vi "fpga_FIFO control (M Class_50Hz).vi"(0 "Time stamp":fxp<+,64,32> format="%.42g", 1 "reset":bool, 2 "filter delay constant":T1=enum."50Hz:10 reporting rate", 5 "Frequency":fxp<+,32,8>, 7 "#ch":fxp<+,5,5>, 9 "PMU VI input valid":bool, 11 "PMU VI output valid":bool) -> (4 "Time Stamp out":fxp<+,64,32> format="%.42g", 14 "data valid?":bool, 15 "Frequency output":fxp<+,32,8> format="%.27g")   [LabVIEW 2013, in "NI_EP_PMU_FPGA.lvlib"]
uses:
  <vilib>/addons/Electrical Power/PMU/NI_EP_PMU_FPGA.lvlib
  <vilib>/addons/Electrical Power/PMU/FPGA/subVIs/fpga_Reporting Rate Configuration.ctl
  <vilib>/rvi/DataTransferAndStorage/Container/Common/niFpgaContainerGetUniqueNameForEmu.vi
  <vilib>/rvi/DataTransferAndStorage/Container/Common/niFpgaContainerSetEmuInfo.vi
  <vilib>/rvi/eio/common/nirviEmuReportErrorAndStop.vi
  <vilib>/rvi/FIFO/Fifo_Resource/nirvififoEmulationWriteFpgaImpl.vi
  <vilib>/rvi/FIFO/Fifo_Resource/nirvififoEmulationReadFpgaImpl.vi
  <vilib>/rvi/LocalResourceManager/LocalResourceManager.xnode
  <vilib>/rvi/DataTransferAndStorage/Container/XNode/niFpgaContainer.xnode
  <vilib>/rvi/FIFO/Fifo_Resource/nirvififoEmulationWrite.vi
  <vilib>/rvi/FXPMathLib/FxpSub/XNode/nifxpmath_Sub.xnode
  <vilib>/rvi/FXPMathLib/basic elements/FxpDiscreteDelay/XNode/nifxpmath_DiscreteDelay.xnode
  <vilib>/rvi/FIFO/Fifo_Resource/nirvififoEmulationRead.vi
  <vilib>/addons/Electrical Power/PQ/Resampling/NI_EP_Resample_FPGA.lvlib
  <vilib>/rvi/FXPMathLib/sim/FxpSim.dll
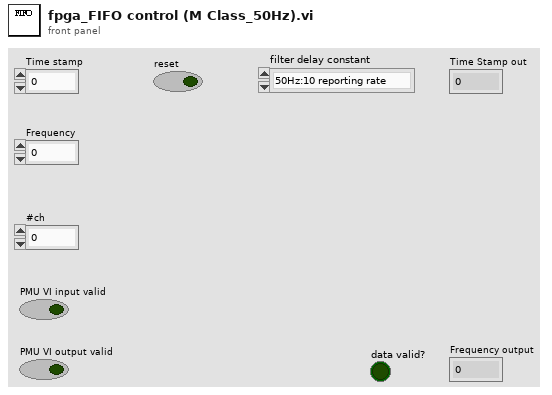
[diagram p1: front panel]
types:
  T1 = typedef "NI_EP_PMU_FPGA.lvlib/fpga_Reporting Rate Configuration.ctl" = enum16{"50Hz:50 reporting rate", "50Hz:25 reporting rate", "50Hz:10 reporting rate", "60Hz:60 reporting rate", "60Hz:30 reporting rate", "60Hz:20 reporting rate", "60Hz:15 reporting rate", "60Hz:12 reporting rate", "60Hz:10 reporting rate"}
  T2 = cluster{"frequency":fxp<+,32,8>, "timestamp":fxp<+,64,32>}
  T3 = cluster{"frequency":fxp<+,32,8>, "timestamp":fxp<+,64,32>}[]
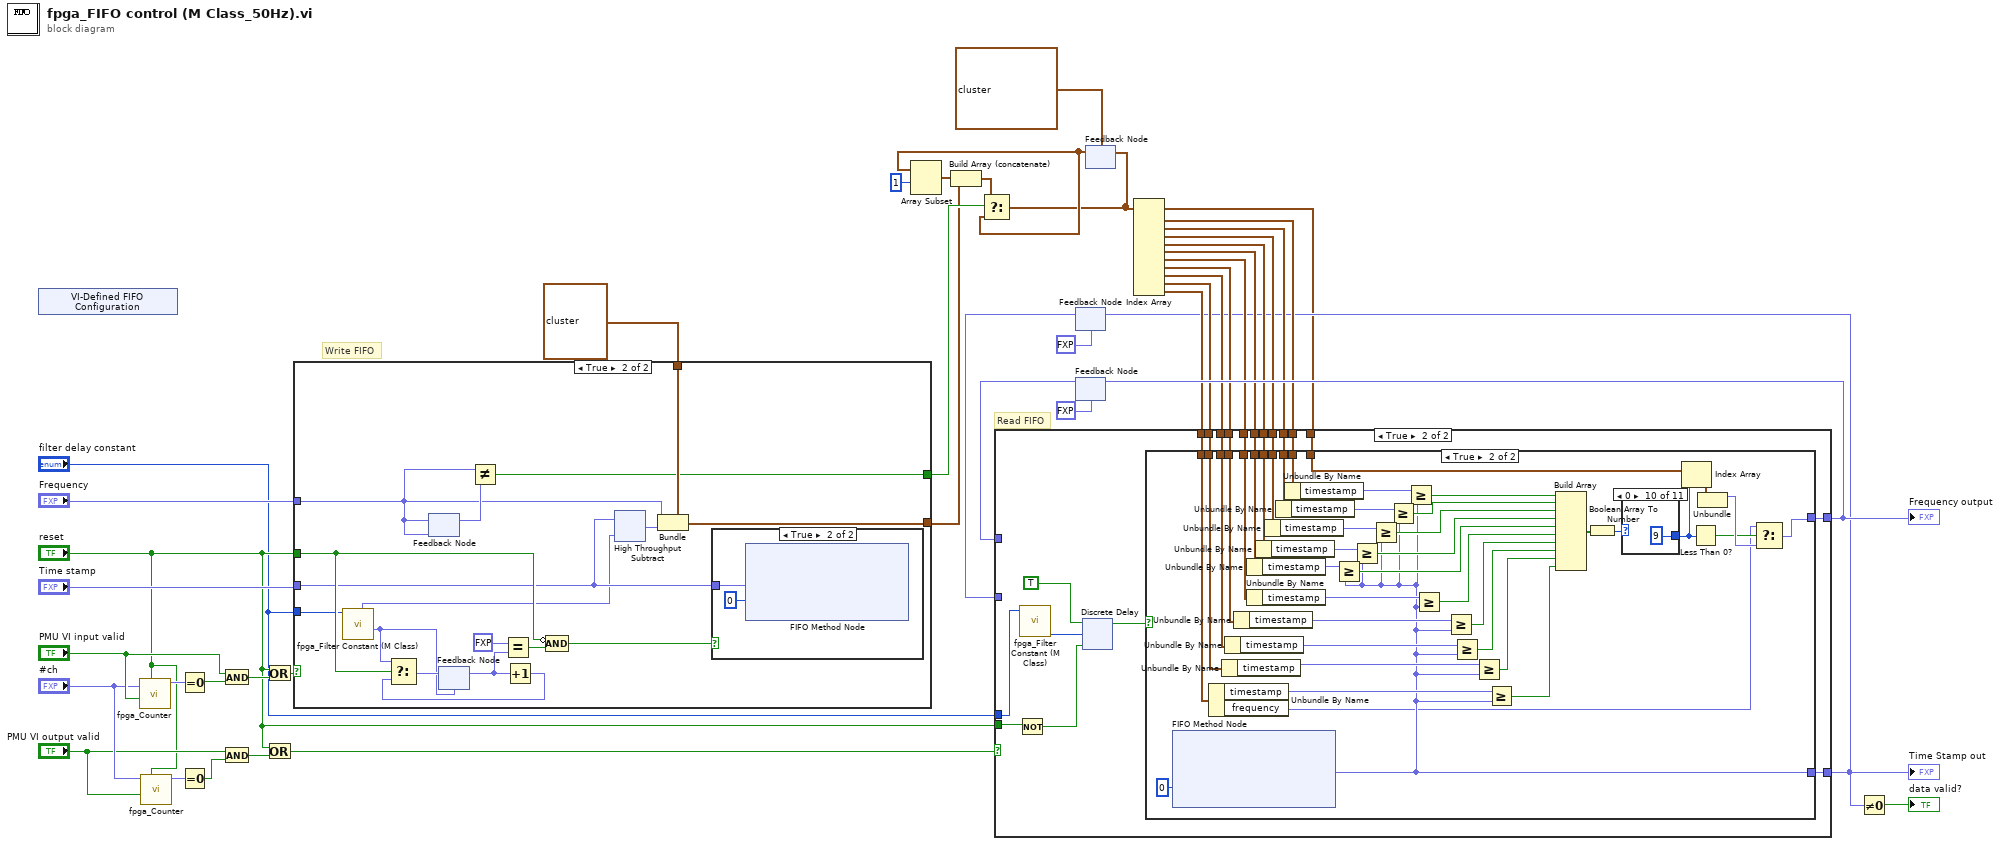
[diagram p0: block diagram]
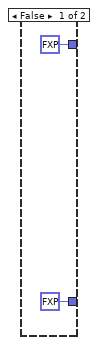
[diagram p3: hidden frame]
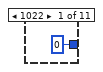
[diagram p4: hidden frame]
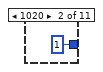
[diagram p5: hidden frame]
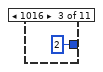
[diagram p6: hidden frame]
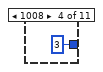
[diagram p7: hidden frame]
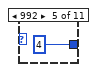
[diagram p8: hidden frame]
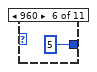
[diagram p9: hidden frame]
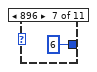
[diagram p10: hidden frame]
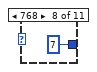
[diagram p11: hidden frame]
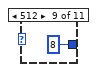
[diagram p12: hidden frame]
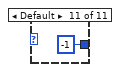
[diagram p13: hidden frame]
diagram:
  # "Read FIFO"
  # "Write FIFO"
  n1 = xnode "VI-Defined FIFO Configuration"() -> ()  [unwired: 1 out]
  n2 = call <vilib>:"fpga_Counter.vi"("reset"="reset", "Input Valid?"="PMU VI input valid", "upper limit"="#ch") -> ("count"=w29:fxp<+,5,5>)  [unwired: 7 in, 1 out]
  n3 = call <vilib>:"fpga_Counter.vi"("reset"="reset", "Input Valid?"="PMU VI output valid", "upper limit"="#ch") -> ("count"=w28:fxp<+,5,5>)  [unwired: 7 in, 1 out]
  n4 = Equal To 0?(x=w29) -> (x = 0?=w40:bool)
  n5 = Equal To 0?(x=w28) -> (x = 0?=w36:bool)
  n6 = And(x="PMU VI input valid", y=w40) -> (x .and. y?=w33:bool)
  n7 = And(x="PMU VI output valid", y=w36) -> (x .and. y?=w39:bool)
  n8 = Or(x="reset", y=w33) -> (x .or. y?=w32:bool)
  n9 = Or(x="reset", y=w39) -> (x .or. y?=w38:bool)
  n10 = case shown="True" w32 {
    tunnel: "Time stamp" -> [_ w44]
    tunnel: "reset" -> [_ w53]
    tunnel: "Frequency" -> [_ w46]
    tunnel: [_ w42] -> w20
    tunnel: [_ w48] -> w19
    tunnel: T2 {"frequency"=0.0, "timestamp"=0.0} -> [_ w47]
    tunnel: "filter delay constant" -> [_ w45]
    frame False {
    }
    frame True {
      n11 = call <vilib>:"fpga_Filter Constant (M Class).vi"("filter delay constant"=w45) -> ("Start"=w52:fxp<+/-,4,4>, "reference delay"=w43:fxp<+,22,0>)  [unwired: 6 in, 3 out]
      n12 = feedback #1(w46) -> (w50:fxp<+,32,8>)
      n13 = feedback-in #1(w46) -> ()
      n14 = feedback #2(w52) -> (w56:fxp<+/-,4,4>)
      n15 = Not Equal?(x=w46, y=w50) -> (x != y?=w42:bool)
      n16 = Equal?(x=fxp<+/-,4,4> 7.0, y=w56) -> (x = y?=w54:bool)
      n17 = Increment(x=w56) -> (x+1=w57:fxp<+,3,3>)
      n18 = Select(t=w52, s=w53, f=w57) -> (s? t:f=w58:fxp<+/-,4,4>)
      n19 = feedback-in #2(w58) -> ()
      n20 = Compound Arithmetic op=AND(invert w53, w54) -> (w51:bool)
      n21 = xnode "High Throughput Subtract"("x"=w44, "y"=w43) -> ("x-y"=w49:fxp<+,64,32>)
      n22 = Bundle(cluster=w47, "frequency"=w46, "timestamp"=w49) -> (w48:T2)
      n23 = case shown="True" w51 {
        tunnel: w44 -> [_ w59]
        frame False {
        }
        frame True {
          n24 = xnode ("FIFO Method Node")("Element"=w59, "Timeout"=0) -> ()  [unwired: 1 in, 2 out]
        }
      }
    }
  }
  n25 = feedback #3(fxp<+,64,32> 0.0 ("Element")) -> (w37:fxp<+,64,32>)
  n26 = feedback #4(fxp<+,32,8> 0.0 ("Element")) -> (w34:fxp<+,32,8>)
  n27 = feedback #5(T3 [{"frequency"=0.0, "timestamp"=0.0}, {"frequency"=0.0, "timestamp"=0.0}, {"frequency"=0.0, "timestamp"=0.0}, {"frequency"=0.0, "timestamp"=0.0}, {"frequency"=0.0, "timestamp"=0.0}, {"frequency"=0.0, "timestamp"=0.0}, {"frequency"=0.0, "timestamp"=0.0}, {"frequency"=0.0, "timestamp"=0.0}, {"frequency"=0.0, "timestamp"=0.0}, {"frequency"=0.0, "timestamp"=0.0}]) -> (w8:T3)
  n28 = Array Subset(array=w8, index=1) -> (w21:T3)  [unwired: 1 in]
  n29 = Build Array (concatenate)(w21, w19) -> (w11:T3)
  n30 = Select(t=w11, s=w20, f=w8) -> (s? t:f=w1:T3)
  n31 = feedback-in #5(w1) -> ()
  n32 = Index Array(array=w1) -> (element #1=w18:T2, element #2=w17:T2, element #3=w16:T2, element #4=w15:T2, element #5=w14:T2, element #6=w10:T2, element #7=w9:T2, element #8=w7:T2, element #9=w6:T2, element #10=w5:T2)  [unwired: 10 in]
  n33 = case shown="True" w38 {
    tunnel: "reset" -> [_ w79]
    tunnel: [w62 w81] -> w3
    tunnel: w37 -> [w62 _]
    tunnel: [w61 w80] -> w24
    tunnel: w34 -> [w61 _]
    tunnel: w18 -> [_ w78]
    tunnel: w17 -> [_ w77]
    tunnel: w16 -> [_ w76]
    tunnel: w15 -> [_ w75]
    tunnel: w14 -> [_ w74]
    tunnel: w1 -> [_ w73]
    tunnel: w10 -> [_ w72]
    tunnel: w9 -> [_ w71]
    tunnel: w7 -> [_ w70]
    tunnel: w6 -> [_ w69]
    tunnel: w5 -> [_ w68]
    tunnel: "filter delay constant" -> [_ w67]
    frame False {
    }
    frame True {
      n34 = Not(x=w79) -> (.not. x?=w65:bool)
      n35 = call <vilib>:"fpga_Filter Constant (M Class).vi"("filter delay constant"=w67) -> ("Total Delay"=w63:u16)  [unwired: 6 in, 4 out]
      n36 = xnode ("Discrete Delay")("D"=TRUE, "n-1[0..511]"=w63, "enable"=w65) -> ("Q"=w66:bool)
      n37 = case shown="True" w66 {
        tunnel: [fxp<+,64,32> 0.0 ("Element") w85] -> w81
        tunnel: [fxp<+,32,8> 0.0 ("frequency") w99] -> w80
        tunnel: w78 -> [_ w119]
        tunnel: w77 -> [_ w120]
        tunnel: w76 -> [_ w121]
        tunnel: w75 -> [_ w122]
        tunnel: w74 -> [_ w123]
        tunnel: w73 -> [_ w86]
        tunnel: w72 -> [_ w106]
        tunnel: w71 -> [_ w103]
        tunnel: w70 -> [_ w97]
        tunnel: w69 -> [_ w96]
        tunnel: w68 -> [_ w95]
        frame False {
        }
        frame True {
          n38 = xnode ("FIFO Method Node")("Timeout"=0) -> ("Element"=w85:fxp<+,64,32>)  [unwired: 1 in, 2 out]
          n39 = Unbundle By Name(w95) -> ("timestamp"=w89:fxp<+,64,32>, "frequency"=w84:fxp<+,32,8>)
          n40 = Unbundle By Name(w96) -> ("timestamp"=w92:fxp<+,64,32>)
          n41 = Unbundle By Name(w97) -> ("timestamp"=w94:fxp<+,64,32>)
          n42 = Unbundle By Name(w103) -> ("timestamp"=w102:fxp<+,64,32>)
          n43 = Unbundle By Name(w123) -> ("timestamp"=w118:fxp<+,64,32>)
          n44 = Unbundle By Name(w106) -> ("timestamp"=w105:fxp<+,64,32>)
          n45 = Unbundle By Name(w122) -> ("timestamp"=w117:fxp<+,64,32>)
          n46 = Unbundle By Name(w121) -> ("timestamp"=w116:fxp<+,64,32>)
          n47 = Unbundle By Name(w120) -> ("timestamp"=w115:fxp<+,64,32>)
          n48 = Unbundle By Name(w119) -> ("timestamp"=w114:fxp<+,64,32>)
          n49 = Greater Or Equal?(x=w118, y=w85) -> (x >= y?=w109:bool)
          n50 = Greater Or Equal?(x=w117, y=w85) -> (x >= y?=w110:bool)
          n51 = Greater Or Equal?(x=w116, y=w85) -> (x >= y?=w111:bool)
          n52 = Greater Or Equal?(x=w115, y=w85) -> (x >= y?=w112:bool)
          n53 = Greater Or Equal?(x=w114, y=w85) -> (x >= y?=w113:bool)
          n54 = Greater Or Equal?(x=w105, y=w85) -> (x >= y?=w104:bool)
          n55 = Greater Or Equal?(x=w102, y=w85) -> (x >= y?=w101:bool)
          n56 = Greater Or Equal?(x=w94, y=w85) -> (x >= y?=w93:bool)
          n57 = Greater Or Equal?(x=w92, y=w85) -> (x >= y?=w91:bool)
          n58 = Greater Or Equal?(x=w89, y=w85) -> (x >= y?=w90:bool)
          n59 = Build Array(w113, w112, w111, w110, w109, w104, w101, w93, w91, w90) -> (w108:bool[])
          n60 = Boolean Array To Number(Boolean array=w108) -> (number=w87:u16)
          n61 = case shown="0" w87 {
            tunnel: [0 ("index") 1 ("index") 2 ("index") 3 ("index") 4 ("index") 5 ("index") 6 ("index") 7 ("index") 8 ("index") 9 ("index") -1 ("index")] -> w88
            frame 1022 {
            }
            frame 1020 {
            }
            frame 1016 {
            }
            frame 1008 {
            }
            frame 992 {
            }
            frame 960 {
            }
            frame 896 {
            }
            frame 768 {
            }
            frame 512 {
            }
            frame 0 {
            }
            frame Default {
            }
          }
          n62 = Index Array(array=w86, index=w88) -> (element=w107:T2)
          n63 = Less Than 0?(x=w88) -> (x < 0?=w98:bool)
          n64 = Unbundle(w107) -> ("frequency"=w100:fxp<+,32,8>)  [unwired: 1 out]
          n65 = Select(t=w84, s=w98, f=w100) -> (s? t:f=w99:fxp<+,32,8>)
        }
      }
    }
  }
  "Time Stamp out" <- w3
  "Frequency output" <- w24
  n66 = feedback-in #3(w3) -> ()
  n67 = feedback-in #4(w24) -> ()
  n68 = Not Equal To 0?(x=w3) -> (x != 0?=→"data valid?":bool)
